vi "Test Update.vi"() -> (3 "value":string)   [LabVIEW 2013]
uses:
  ACNET Monitor.lvlib
panel:
  in  "XML File Path":path=path "C:/Users/plane/Documents/acnet_monitor_config_from_acnetize.xml"
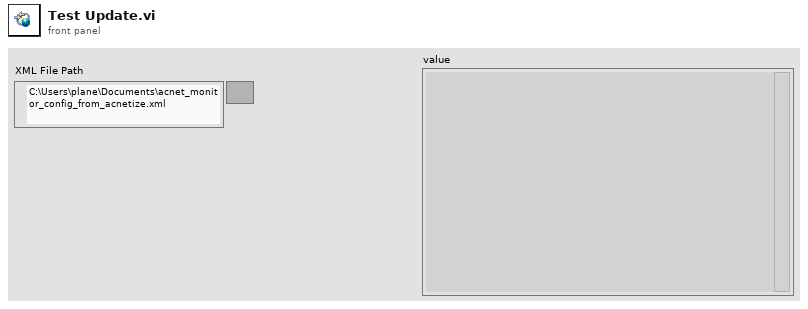
[diagram p1: front panel]
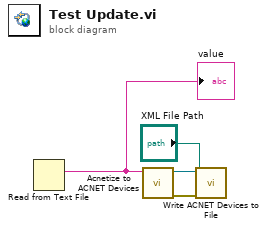
[diagram p0: block diagram]
diagram:
  n1 = Read from Text File() -> (text=w1:string)  [unwired: 4 in, 3 out]
  "value" <- w1
  n2 = call "Acnetize to ACNET Devices.vi"("Acnetize Configuration"=w1) -> ("error out"=w3:errorcluster, "ACNET Devices"=w4:refnum<class "ACNET Devices.lvclass">)  [unwired: 9 in]
  n3 = call "Write ACNET Devices to File.vi"("error in (no error)"=w3, "XML File Path"="XML File Path", "ACNET Devices in"=w4) -> ()  [unwired: 7 in, 2 out]
